vi "FRD-conv_freq-unit.vi"(6 "Frequency Unit":enum16{"Hz", "rad/s"}(ring), 11 "FRD-model":T1) -> (3 "FRD-out":T1)   [LabVIEW 2017]
uses:
  controls/FrdData.ctl
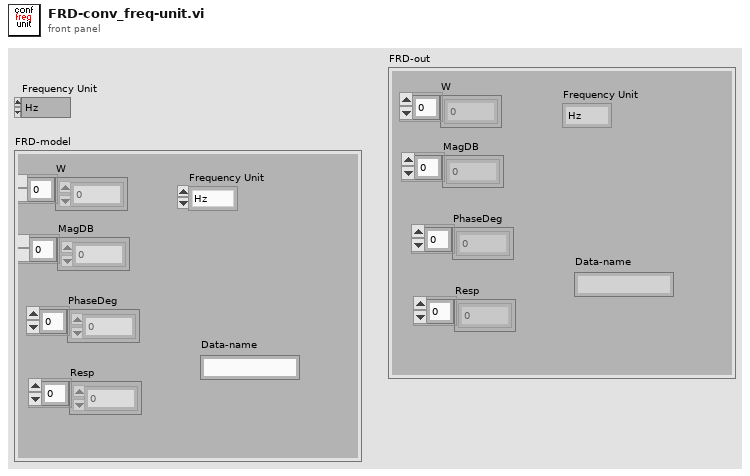
[diagram p1: front panel]
types:
  T1 = typedef "FrdData.ctl" = cluster{"Frequency Unit":enum16{"Hz", "rad/s"}, "W":dbl[], "MagDB":dbl[], "PhaseDeg":dbl[], "Resp":cdb[], "Data-name":string}
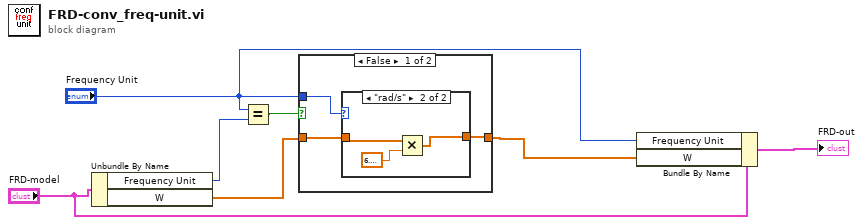
[diagram p0: block diagram]
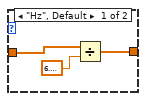
[diagram p2: hidden frame]
diagram:
  n1 = Unbundle By Name("FRD-model") -> ("Frequency Unit"=w5:enum16{"Hz", "rad/s"}, "W"=w7:dbl[])
  n2 = Equal?(x="Frequency Unit", y=w5) -> (x = y?=w6:bool)
  n3 = case shown="False" w6 {
    tunnel: w7 -> [w9 w17]
    tunnel: [w8 w17] -> w3
    tunnel: "Frequency Unit" -> [w10 _]
    frame False {
      n4 = case shown="\"rad/s\"" w10 {
        tunnel: w9 -> [w11 w14]
        tunnel: [w12 w15] -> w8
        frame "Hz", Default {
          n5 = Divide(x=w11, y=6.283185307179586) -> (x/y=w12:dbl[])
        }
        frame "rad/s" {
          n6 = Multiply(x=w14, y=6.283185307179586) -> (x*y=w15:dbl[])
        }
      }
    }
    frame True {
    }
  }
  n7 = Bundle By Name(cluster="FRD-model", "Frequency Unit"="Frequency Unit", "W"=w3) -> (→"FRD-out":T1)
